vi "Launch Syringe Stepper Actor.vi"(5 "DedicatedEnQrs":refnum<queue>, 7 "Name":string="Stepper", 8 "error in (no error)":errorcluster, 9 "Syringe Pressure StateQ":refnum<queue>, 10 "Interlock Chain":refnum<class "Interlock Chain.lvclass">, 11 "Caller Actor in":refnum<class "Actor.lvclass">) -> (0 "error out":errorcluster, 3 "Caller-To-Actor Enqueuer":refnum<class "Message Enqueuer.lvclass">)   [LabVIEW 2015, in "Stepper.lvclass"]
uses:
  Stepper.lvclass
  <vilib>/ActorFramework/Message Enqueuer/Message Enqueuer.lvclass
  Interlocks/Interlock Chain/Interlock Chain.lvclass
  <vilib>/ActorFramework/Actor/Actor.lvclass
  Controls/Dedicated Enqueuers.ctl
  Controls/Vacuum State Cluster.ctl
  Controls/Vacuum State Enumerator.ctl
  CO2 Actor/CO2 Actor.lvclass
  Stepper.lvclass/Stepper.ctl
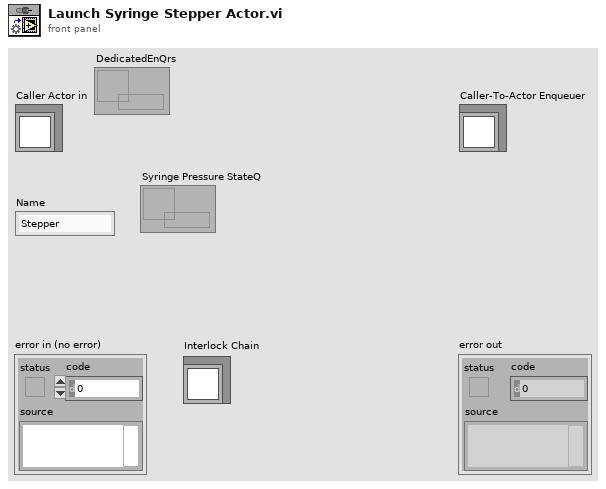
[diagram p1: front panel]
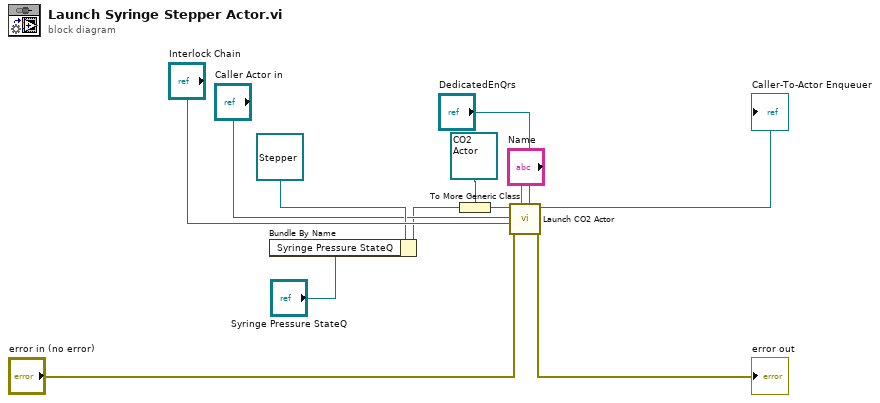
[diagram p0: block diagram]
diagram:
  n1 = Bundle By Name(cluster=refnum<class "Stepper.lvclass"> refnum ("Stepper in"), "Syringe Pressure StateQ"="Syringe Pressure StateQ") -> (w2:refnum<class "Stepper.lvclass">)
  n2 = To More Generic Class(target class=refnum<class "CO2 Actor.lvclass"> refnum ("CO2 Actor in"), reference=w2) -> (generic class reference=w5:refnum<class "CO2 Actor.lvclass">)
  n3 = call "Launch CO2 Actor.vi"("DedicatedEnQrs"="DedicatedEnQrs", "Name"="Name", "error in (no error)"="error in (no error)", "Interlock Chain"="Interlock Chain", "Caller Actor in"="Caller Actor in", "CO2 Actor in"=w5) -> ("error out"=→"error out":errorcluster, "Caller-To-Actor Enqueuer"=→"Caller-To-Actor Enqueuer":refnum<class "Message Enqueuer.lvclass">)  [unwired: 4 in]
